vi "Parse Core.vi"(8 "error in (no error)":errorcluster, 11 "Config Parser SPI_3W in":refnum<class "Config Parser SPI_3W.lvclass">) -> (0 "error out":errorcluster, 2 "Config Array":string[](array[string]), 3 "Config Parser SPI_3W out":refnum<class "Config Parser SPI_3W.lvclass">)   [LabVIEW 2018, in "Config Parser SPI_3W.lvlib" / "Config Parser SPI_3W.lvclass"]
uses:
  Config Parser SPI_3W.lvclass
  C:/P4 Workspace/PC Client/Solutions/5g_eap/trunk/1.0/HiSi5GmmWave/Pattern_Gen_Tool/Interfaces/File Parser Interface.lvlibp/Interfaces/File Parser Interface/File Parser Interface.lvclass
  Interfaces/File Parser Interface.lvlibp/Interfaces/File Parser Interface/Read File Path.vi
  <vilib>/Utility/file.llb/Read Delimited Spreadsheet (string).vi
  Interfaces/File Parser Interface.lvlibp/Interfaces/File Parser Interface/File Parser Interface.lvclass
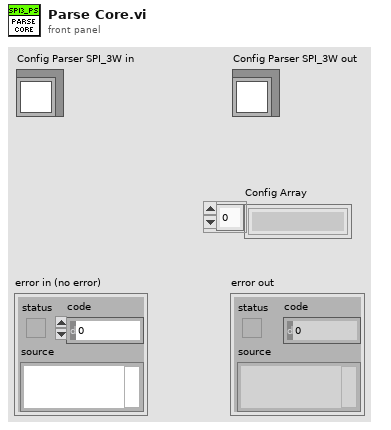
[diagram p1: front panel]
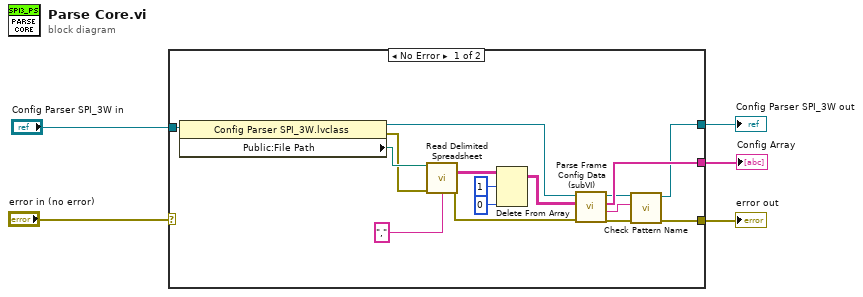
[diagram p0: block diagram]
diagram:
  n1 = case shown="No Error" "error in (no error)" {
    selector: "error in (no error)" -> [_ w22]
    tunnel: "Config Parser SPI_3W in" -> [w16 w23]
    tunnel: [w9 w23] -> w3
    tunnel: [w13 _] -> w2
    tunnel: [w11 w22] -> w1
    frame No Error {
      n2 = property class="Config Parser SPI_3W.lvclass"(reference=w16) -> (reference out=w14:refnum<class "Config Parser SPI_3W.lvclass">, error out=w7:errorcluster, "Public:File Path"=w18:path)  [unwired: 1 in]
      n3 = call-poly <vilib>:"Read Delimited Spreadsheet.vi"("file path (dialog if empty)"=w18, "error in (no error)"=w7, "delimiter (\\t)"="," ("delimiter (\\t)")) -> ("all rows"=w21:string[][], "error out"=w6:errorcluster)  [unwired: 7 in, 4 out]
      n4 = Delete From Array(array=w21, length=1, index (row)=0) -> (array with subset deleted=w15:string[][])  [unwired: 1 in, 1 out]
      n5 = call-dynamic "Parse Frame Config Data (subVI).vi"("error in (no error)"=w6, "CSV Raw Data"=w15, "Config Parser SPI_3W in"=w14) -> ("error out"=w12:errorcluster, "Pattern Name out"=w8:string, "Config Data out"=w13:string[], "Config Parser SPI_3W out"=w10:refnum<class "Config Parser SPI_3W.lvclass">)  [unwired: 5 in]
      n6 = call "Check Pattern Name.vi"("error in (no error)"=w12, "Pattern Name"=w8, "File Parser Interface in"=w10) -> ("error out"=w11:errorcluster, "File Parser Interface out"=w9:refnum<class "Config Parser SPI_3W.lvclass">)  [unwired: 7 in]
    }
    frame Error {
    }
  }
  "error out" <- w1
  "Config Parser SPI_3W out" <- w3
  "Config Array" <- w2
